vi "Exercise3BTS.vi"() -> ()   [LabVIEW 2014]
uses:
  <vilib>/Utility/file.llb/Write To Spreadsheet File (DBL).vi
panel:
  out "Delay Time  (Sec)":dbl
  out "Reaction Time":dbl
  in  "stop":bool
  in  "Start":bool
  out "LED":bool
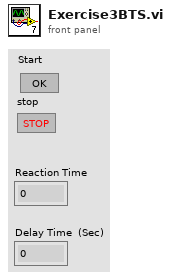
[diagram p1: front panel]
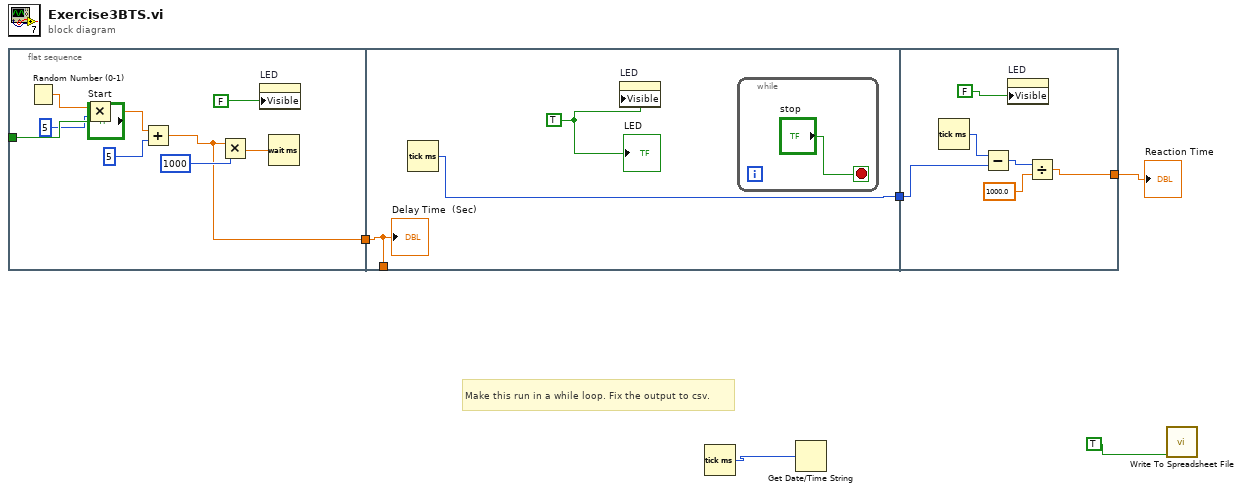
[diagram p0: block diagram]
diagram:
  # "Make this run in a while loop. Fix the output to csv."
  n1 = flat-sequence {
    tunnel: "Start" -> [_]
    tunnel: [w7] -> w3
    tunnel: [w17] -> w5
    tunnel: w3 -> [w15]
    tunnel: [w15] -> _
    tunnel: [w21] -> w4
    tunnel: w5 -> [w20]
    frame #0 {
      n2 = Random Number (0-1)() -> (number: 0 to 1=w10:dbl)
      n3 = Multiply(x=w10, y=5) -> (x*y=w13:dbl)
      n4 = Add(x=w13, y=5) -> (x+y=w7:dbl)
      n5 = Multiply(x=w7, y=1000) -> (x*y=w8:dbl)
      n6 = property on="LED" class="Bool (strict)"("Visible"=FALSE) -> ()  [unwired: 2 in, 2 out]
      n7 = Wait (ms)(milliseconds to wait=w8) -> ()  [unwired: 1 out]
    }
    frame #1 {
      w16 = TRUE
      n8 = Tick Count (ms)() -> (millisecond timer value=w17:u32)
      n9 = property on="LED" class="Bool (strict)"("Visible"=w16) -> ()  [unwired: 2 in, 2 out]
      n10 = while {
        stop <- "stop" stop-if-true
      }
      "LED" <- w16
      "Delay Time  (Sec)" <- w15
    }
    frame #2 {
      n11 = Tick Count (ms)() -> (millisecond timer value=w24:u32)
      n12 = Subtract(x=w24, y=w20) -> (x-y=w23:u32)
      n13 = property on="LED" class="Bool (strict)"("Visible"=FALSE) -> ()  [unwired: 2 in, 2 out]
      n14 = Divide(x=w23, y=1000.0) -> (x/y=w21:dbl)
    }
  }
  n15 = Tick Count (ms)() -> (millisecond timer value=w1:u32)
  n16 = Get Date/Time String(seconds (now)=w1) -> ()  [unwired: 2 in, 2 out]
  n17 = call-poly <vilib>:"Write To Spreadsheet File.vi"("append to file? (new file:F)"=TRUE) -> ()  [unwired: 7 in, 1 out]
  "Reaction Time" <- w4
